vi "Init.vi"(5 "Instrument.lvclass 2":refnum<class "Instrument.lvclass">, 6 "Step":dbl, 7 "Instrument 1.lvclass":refnum<class "Instrument.lvclass">, 8 "error in (no error)":errorcluster, 9 "Max":dbl, 10 "Init":dbl, 11 "Measurement1D in":refnum<class "RT_meas.lvclass">) -> (0 "error out":errorcluster, 3 "Measurement1D out":refnum<class "RT_meas.lvclass">)   [LabVIEW 2014, in "RT_meas.lvclass"]
uses:
  RT_meas.lvclass
  Abstract/Measurement/Measurement2D/Measurement2D.lvclass
  Abstract/Instrument/Instrument/Instrument.lvclass
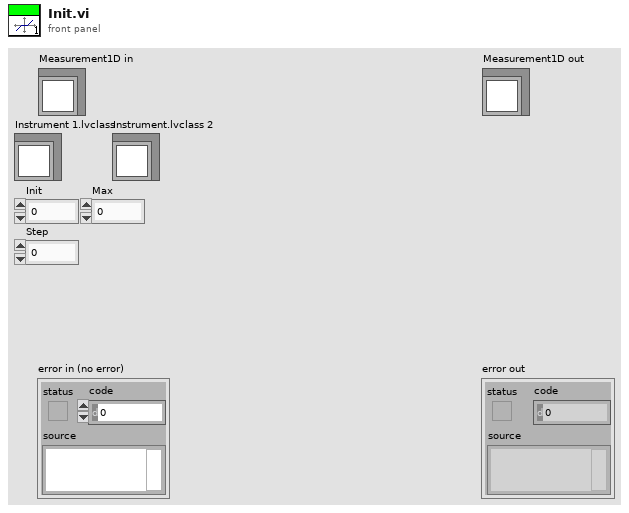
[diagram p1: front panel]
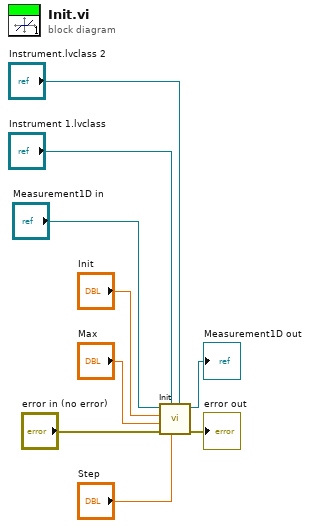
[diagram p0: block diagram]
diagram:
  n1 = call-parent "Init.vi"("Instrument.lvclass 2"="Instrument.lvclass 2", "Step"="Step", "Instrument 1.lvclass"="Instrument 1.lvclass", "error in (no error)"="error in (no error)", "Max"="Max", "Init"="Init", "Measurement1D in"="Measurement1D in") -> ("error out"=→"error out":errorcluster, "Measurement1D out"=→"Measurement1D out":refnum<class "RT_meas.lvclass">)  [unwired: 3 in]
